vi "charTest.vi"() -> ()   [LabVIEW 2025]
panel:
  out "Numeric":i32
  out "element":i32
  out "size(s) 4":i32
  out "size(s) 3":i32
  out "size(s) 2":i32[](array[numeric])
  in  "Array":string[](array[string])
  out "size(s)":i32
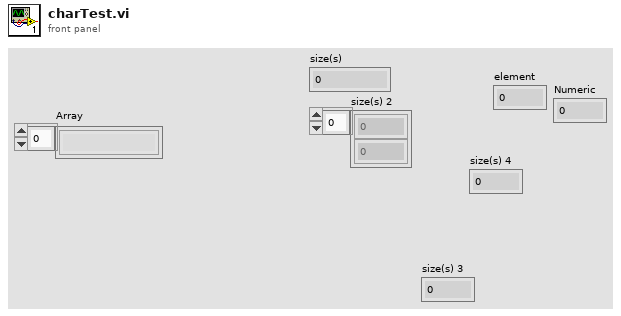
[diagram p1: front panel]
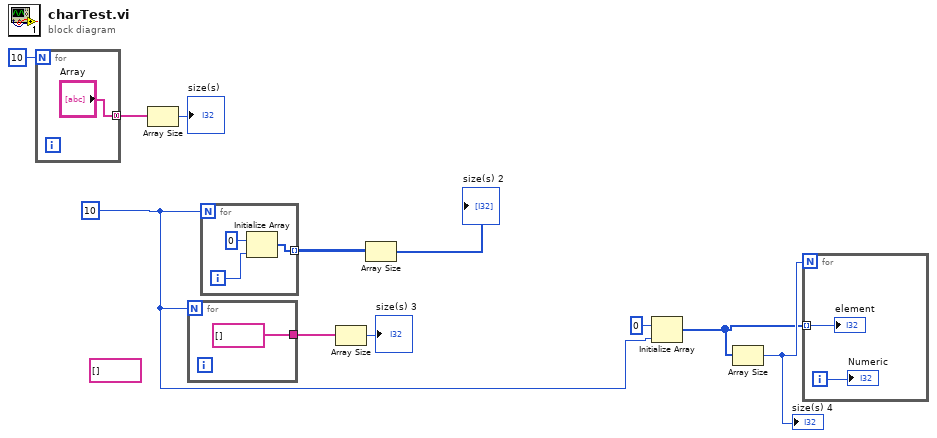
[diagram p0: block diagram]
diagram:
  (unwired) string[] []
  w3 = 10
  n1 = for {
    N: 10 -> [_]
    tunnel: ["Array"] -> w9 mode=concatenating
  }
  n2 = Array Size(array=w9) -> (size(s)=→"size(s)":i32)
  n3 = for {
    N: w3 -> [_]
    tunnel: [string[] []] -> w7
  }
  n4 = for {
    N: w3 -> [_]
    tunnel: [w15] -> w5 mode=indexing
    i -> [w14]
    n5 = Initialize Array(0 ("element"), w14) -> (w15:i32[])
  }
  n6 = Array Size(array=w7) -> (size(s)=→"size(s) 3":i32)
  n7 = Array Size(array=w5) -> (size(s)=→"size(s) 2":i32[])
  n8 = Initialize Array(0 ("element"), w3) -> (w1:i32[])
  n9 = Array Size(array=w1) -> (size(s)=w2:i32)
  "size(s) 4" <- w2
  n10 = for {
    N: w2 -> [_]
    tunnel: w1 -> [w18] mode=indexing
    i -> [w17]
    "element" <- w18
    "Numeric" <- w17
  }
